vi "calibrationSpectrometer_getSample_Timestamp.vi"(8 "error in (no error)":errorcluster, 11 "Timestamp_Ctl":T1) -> (0 "error out":errorcluster, 2 "function return":i32, 3 "Timestamp_Ctl out":T1)   [LabVIEW 2016, in "SALLV_calibrationSpectrometer.lvlib"]
doc: "int calibrationSpectrometer_shm_getSample_TimestampLV(calibrationSpectrometer_TimestampLV *Timestamp_Ctl );"
uses:
  SALLV_calibrationSpectrometer.lvlib
  DataTypes/Timestamp.ctl
  SALLV_calibrationSpectrometer.so
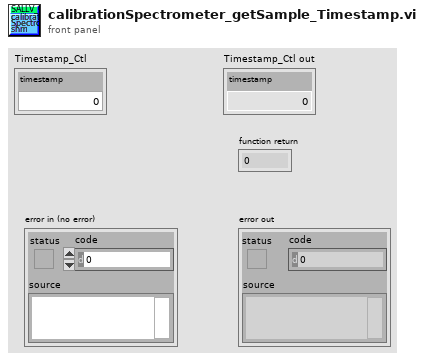
[diagram p1: front panel]
types:
  T1 = typedef "SALLV_calibrationSpectrometer.lvlib/Timestamp.ctl" = cluster{"timestamp":dbl}
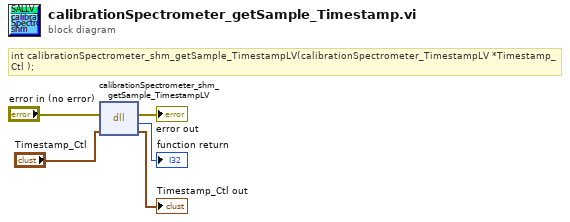
[diagram p0: block diagram]
diagram:
  # "int calibrationSpectrometer_shm_getSample_TimestampLV(calibrationSpectrometer_TimestampLV *Timestamp_Ctl );"
  n1 = dll-call lib="home/harini/TCS/sallv_sedspectrometer/SALLV_calibrationSpectrometer.*" fn="calibrationSpectrometer_shm_getSample_TimestampLV"(error in="error in (no error)", "Timestamp_Ctl"="Timestamp_Ctl") -> (error out=→"error out":errorcluster, →"function return":i32, "Timestamp_Ctl"=→"Timestamp_Ctl out":T1)  [unwired: 2 in, 1 out]
